vi "AnalyseLV.vi"(8 "error in (no error)":errorcluster, 10 "ImageData":T2, 11 "FluorescenceAnalyser in":refnum<class "FluorescenceAnalyser.lvclass">) -> (0 "error out":errorcluster, 3 "FluorescenceAnalyser out":refnum<class "FluorescenceAnalyser.lvclass">)   [LabVIEW 2011, in "Tools.lvlib" / "Imaging.lvlib" / "FluorescenceAnalyser.lvclass"]
uses:
  FluorescenceAnalyser.lvclass
  <vilib>/Analysis/NI_AALBase.lvlib
  ImageAnalyser.lvclass
  Imaging.lvlib
panel:
  in  "detuning MHz":dbl
  out "Image":T1(plugin-control)
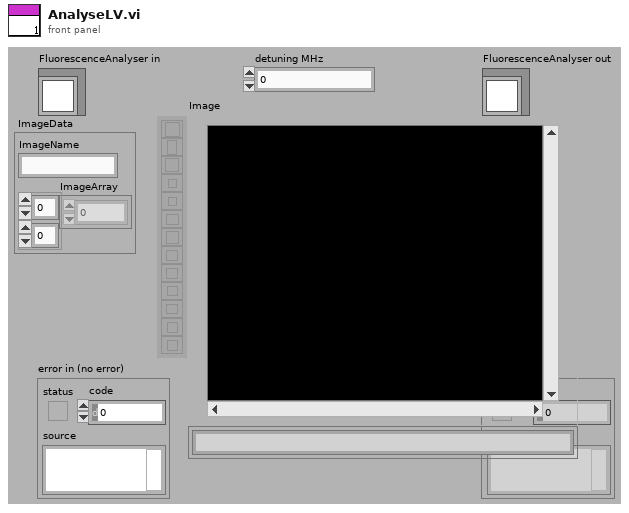
[diagram p1: front panel]
types:
  T1 = typedef "IMAQ Image.ctl" = refnum<image>
  T2 = cluster{"ImageName":string, "ImageArray":sgl[][]}
  T3 = typedef "IMAQ Rectangle" = cluster{"Left":i32, "Top":i32, "Right":i32, "Bottom":i32, "Rotation":dbl}
  T4 = cluster{"Name":string, "Results":dbl[], "AnalysisType":string}
  T5 = cluster{"Objects":u16, "Threshold":i32, "Reject Border":bool, "Fill Holes":bool, "Min Object Size":bool, "Min Size":i32, "Max Object Size":bool, "Max Size":i32, "Show Search Area":bool, "Show Center":bool, "Show Bounding Box":bool}
  T6 = typedef "Image Type" = u32
  T7 = cluster{"Left":i32, "Top":i32, "Right":i32, "Bottom":i32}
  T8 = cluster{"Object Center":cluster{"X":sgl, "Y":sgl}, "Bounding Box":cluster{"X Left":i32, "Y Top":i32, "X Right":i32, "Y Bottom":i32}, "Area":sgl, "Orientation":sgl, "Aspect Ratio":sgl, "Nb Holes":i32}[]
  T9 = cluster{"Object Center":cluster{"X":sgl, "Y":sgl}, "Bounding Box":cluster{"X Left":i32, "Y Top":i32, "X Right":i32, "Y Bottom":i32}, "Area":sgl, "Orientation":sgl, "Aspect Ratio":sgl, "Nb Holes":i32}
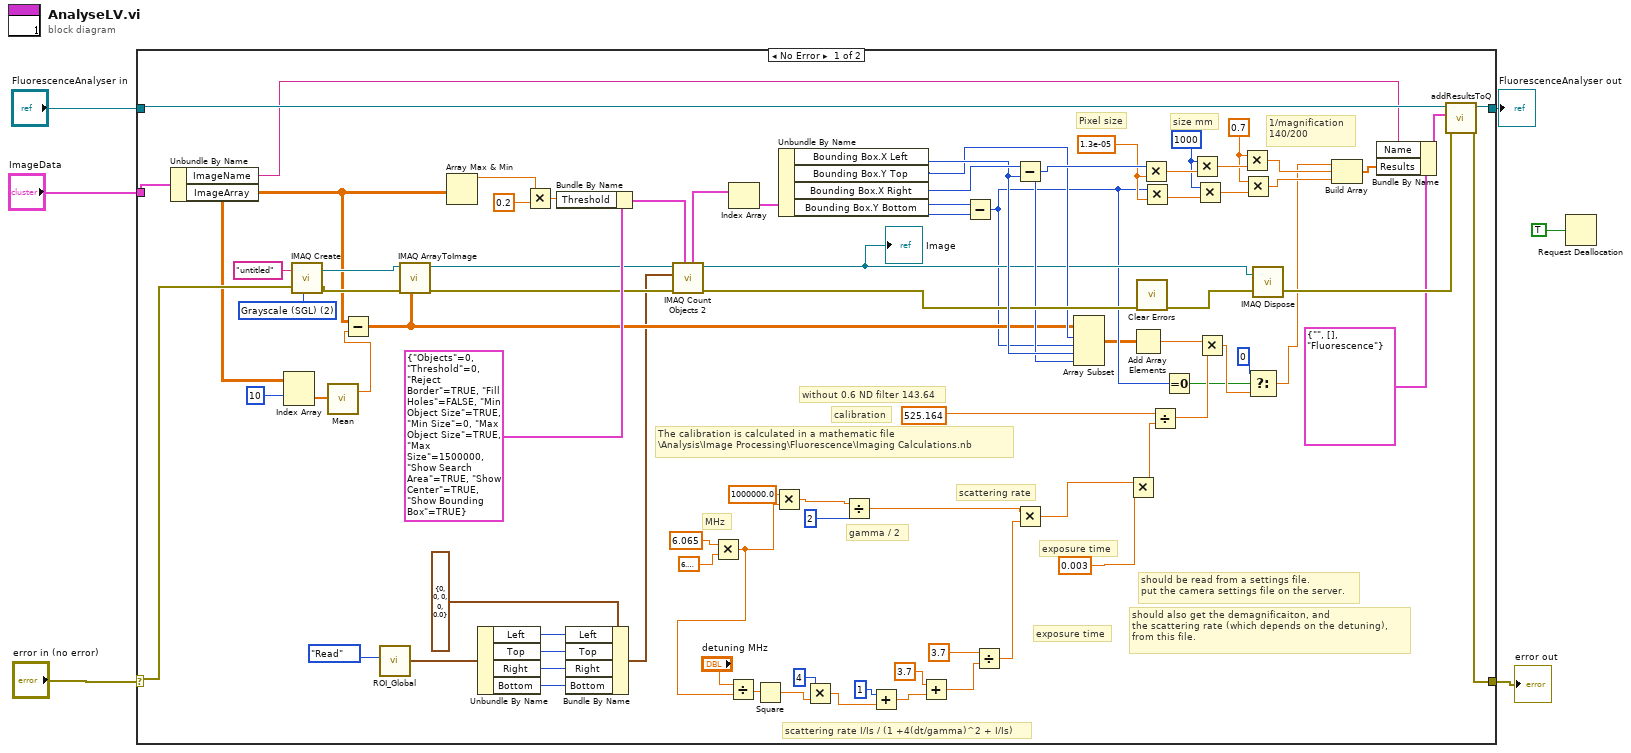
[diagram p0: block diagram]
diagram:
  n1 = case shown="No Error" "error in (no error)" {
    selector: "error in (no error)" -> [w72 w91]
    tunnel: [w60 w91] -> w5
    tunnel: [w62 w90] -> w3
    tunnel: "FluorescenceAnalyser in" -> [w61 w90]
    tunnel: "ImageData" -> [w89 _]
    frame No Error {
      w42 = 0.7
      w55 = 1000
      w70 = 1.3e-05
      w74 = T6 2 items=["Grayscale (U8)", "Grayscale (I16)", "Grayscale (SGL)", "Complex (CSG)", "RGB (U32)", "HSL (U32)", "RGB (U64)", "Grayscale (U16)"] ("Image Type")
      # "gamma / 2"
      # "scattering rate I/Is / (1 +4(dt/gamma)^2 + I/Is)"
      # "MHz"
      # "exposure time"
      # "without 0.6 ND filter 143.64"
      # "Pixel size"
      # "should also get the demagnificaiton, and\nthe scattering rate (which depends on the detuning),\nfrom this file."
      # "should be read from a settings file.\nput the camera settings file on the server."
      # "The calibration is calculated in a mathematic file\n\\Analysis\\Image Processing\\Fluorescence\\Imaging Calculations.nb"
      # "1/magnification\n140/200"
      # "size mm"
      # "exposure time"
      # "scattering rate"
      # "calibration"
      n2 = Unbundle By Name(w89) -> ("ImageName"=w48:string, "ImageArray"=w51:sgl[][])
      n3 = Index Array(array=w51, index (row)=10) -> (element=w68:sgl[])  [unwired: 1 in]
      n4 = call "IMAQ Create"("Image Name"="untitled", "Image Type"=w74, "error in (no error)"=w72) -> ("New Image"=w88:T1, "error out"=w87:errorcluster)  [unwired: 2 in]
      n5 = call <vilib>:"Mean.vi"("X"=w68) -> ("mean"=w37:dbl)  [unwired: 1 out]
      n6 = Subtract(x=w51, y=w37) -> (x-y=w41:dbl[][])
      n7 = call "ROI_Global.vi"("Action"=enum16{"Write", "Read"}."Read") -> ("ROI"=w31:T7)  [unwired: 10 in]
      n8 = call "IMAQ ArrayToImage"("Image Pixels (Float)"=w41, "error in (no error)"=w87, "Image"=w88) -> ("error out"=w79:errorcluster, "Image Out"=w80:T1)  [unwired: 7 in]
      n9 = Array Max & Min(array=w51) -> (max value=w83:sgl)  [unwired: 3 out]
      n10 = Unbundle By Name(w31) -> ("Left"=w30:i32, "Top"=w29:i32, "Right"=w28:i32, "Bottom"=w27:i32)
      n11 = Multiply(x=w83, y=0.2) -> (x*y=w84:dbl)
      n12 = Bundle By Name(cluster=T5 {"Objects"=0, "Threshold"=0, "Reject Border"=TRUE, "Fill Holes"=FALSE, "Min Object Size"=TRUE, "Min Size"=0, "Max Object Size"=TRUE, "Max Size"=1500000, "Show Search Area"=TRUE, "Show Center"=TRUE, "Show Bounding Box"=TRUE} ("Settings"), "Threshold"=w84) -> (w81:T5)
      n13 = Bundle By Name(cluster=T3 {"Left"=0, "Top"=0, "Right"=0, "Bottom"=0, "Rotation"=0.0} ("Search Rect (entire image)"), "Left"=w30, "Top"=w29, "Right"=w28, "Bottom"=w27) -> (w26:T3)
      n14 = call "IMAQ Count Objects 2"("Settings"=w81, "error in (no error)"=w79, "Search Rect (entire image)"=w26, "Image"=w80) -> ("error out"=w73:errorcluster, "Image Out"=w54:T1, "Objects"=w78:T8)  [unwired: 3 in, 2 out]
      "Image" <- w54
      n15 = Multiply(x=6.065, y=6.283185307179586) -> (x*y=w16:dbl)
      n16 = Divide(x="detuning MHz", y=w16) -> (x/y=w15:dbl)
      n17 = Index Array(array=w78) -> (element=w77:T9)  [unwired: 1 in]
      n18 = Square(x=w15) -> (x^2=w14:dbl)
      n19 = Multiply(x=1000000.0, y=w16) -> (x*y=w22:dbl)
      n20 = Unbundle By Name(w77) -> ("Bounding Box.X Left"=w75:i32, "Bounding Box.Y Top"=w58:i32, "Bounding Box.X Right"=w76:i32, "Bounding Box.Y Bottom"=w59:i32)
      n21 = Multiply(x=4, y=w14) -> (x*y=w13:dbl)
      n22 = Divide(x=w22, y=2) -> (x/y=w9:dbl)
      n23 = Add(x=1, y=w13) -> (x+y=w12:dbl)
      n24 = Add(x=3.7, y=w12) -> (x+y=w10:dbl)
      n25 = Subtract(x=w59, y=w58) -> (x-y=w36:i32)
      n26 = Divide(x=3.7, y=w10) -> (x/y=w8:dbl)
      n27 = Subtract(x=w76, y=w75) -> (x-y=w71:i32)
      n28 = Multiply(x=w9, y=w8) -> (x*y=w7:dbl)
      n29 = Array Subset(array=w41, index (row)=w58, length (row)=w36, index (col)=w75, length (col)=w71) -> (w34:dbl[][])
      n30 = Multiply(x=w7, y=0.003) -> (x*y=w66:dbl)
      n31 = Add Array Elements(numeric array=w34) -> (sum=w64:dbl)
      n32 = call <vilib>:"Clear Errors.vi"("error in (no error)"=w73) -> ("error out"=w53:errorcluster)  [unwired: 6 in]
      n33 = Multiply(x=w71, y=w70) -> (x*y=w57:dbl)
      n34 = Multiply(x=w36, y=w70) -> (x*y=w56:dbl)
      n35 = Divide(x=525.164, y=w66) -> (x/y=w63:dbl)
      n36 = Equal To 0?(x=w36) -> (x = 0?=w35:bool)
      n37 = Multiply(x=w55, y=w57) -> (x*y=w46:dbl)
      n38 = Multiply(x=w55, y=w56) -> (x*y=w45:dbl)
      n39 = Multiply(x=w64, y=w63) -> (x*y=w39:dbl)
      n40 = Multiply(x=w42, y=w46) -> (x*y=w44:dbl)
      n41 = Multiply(x=w42, y=w45) -> (x*y=w43:dbl)
      n42 = Select(t=0, s=w35, f=w39) -> (s? t:f=w38:dbl)
      n43 = call "IMAQ Dispose"("Image"=w54, "error in (no error)"=w53) -> ("error out"=w52:errorcluster)  [unwired: 4 in]
      n44 = Build Array(w38, w44, w43) -> (w49:dbl[])
      n45 = Bundle By Name(cluster=T4 {"Name"="", "Results"=[], "AnalysisType"="Fluorescence"} ("output cluster"), "Name"=w48, "Results"=w49) -> (w47:T4)
      n46 = call "addResultsToQ.vi"("error in (no error)"=w52, "Results"=w47, "ImageAnalyser in"=w61) -> ("error out"=w60:errorcluster, "ImageAnalyser out"=w62:refnum<class "FluorescenceAnalyser.lvclass">)  [unwired: 7 in]
    }
    frame Error {
    }
  }
  "error out" <- w5
  "FluorescenceAnalyser out" <- w3
  n47 = Request Deallocation(TRUE ("flag")) -> ()
